vi "Set Tree Symbols.vi"(8 "error in (no error)":errorcluster, 11 "File Explorer in":refnum<class "File Explorer.lvclass">) -> (0 "error out":errorcluster, 3 "File Explorer out":refnum<class "File Explorer.lvclass">)   [LabVIEW 2019, in "File Explorer.lvlib" / "File Explorer.lvclass"]
uses:
  <vilib>/gpm_packages/@cs/file-explorer-extension/Source/File Explorer/File Explorer/File Explorer.lvclass
  <vilib>/gpm_packages/@cs/file-explorer-extension/Source/File Explorer/File Explorer/File Explorer.lvclass/File Explorer.ctl
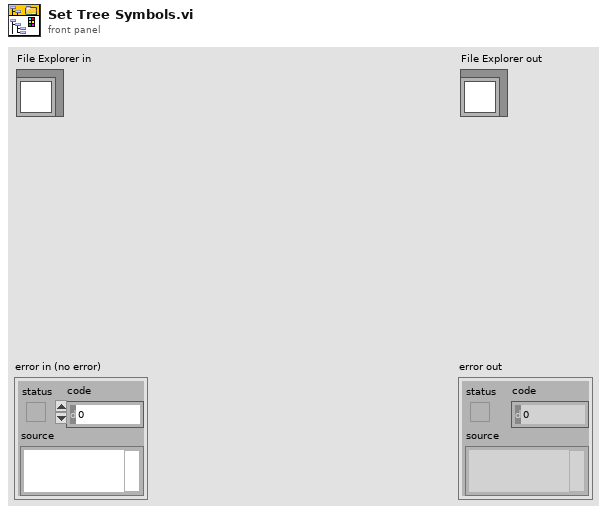
[diagram p1: front panel]
types:
  T1 = typedef "imagedata.ctl" = cluster{"image type":i32, "image depth":i32, "image":u8[], "mask":u8[], "colors":u32[], "Rectangle":cluster{"left":i16, "top":i16, "right":i16, "bottom":i16}}
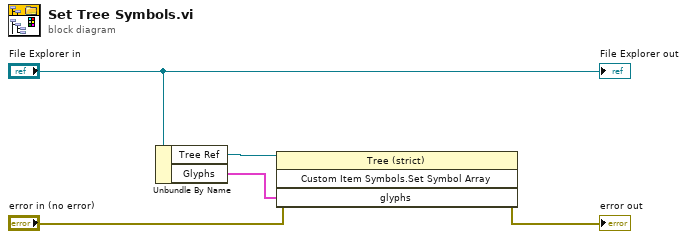
[diagram p0: block diagram]
diagram:
  n1 = Unbundle By Name("File Explorer in") -> ("Tree Ref"=w4:refnum<vi>, "Glyphs"=w3:T1[])
  n2 = invoke class="Tree (strict)" method="Custom Item Symbols.Set Symbol Array"(reference=w4, error in="error in (no error)", "glyphs"=w3) -> (error out=→"error out":errorcluster)  [unwired: 1 in, 3 out]
  "File Explorer out" <- "File Explorer in"
